vi "Setup.vi"(8 "error in (no error)":errorcluster, 11 "Setup Error In":refnum<class "Setup Error.lvclass">) -> (0 "error out":errorcluster, 3 "Setup Error Out":refnum<class "Setup Error.lvclass">)   [LabVIEW 2020, in "Setup Error.lvclass"]
doc: "Setup method called by the testing framework to set up test fixture before each test method is called."
uses:
  Setup Error.lvclass
  source/LUnit Test Case.lvclass
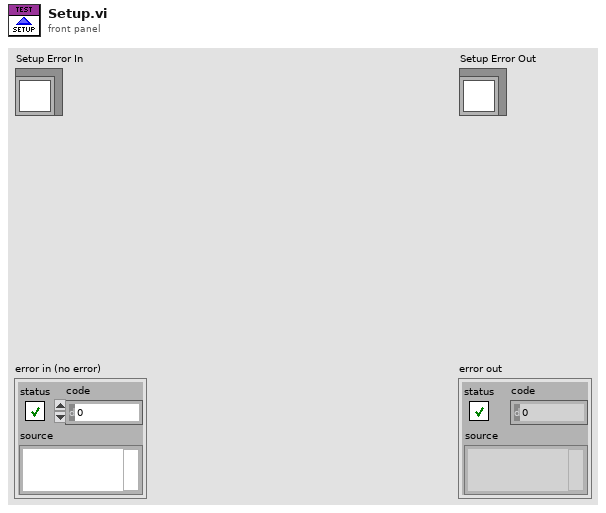
[diagram p1: front panel]
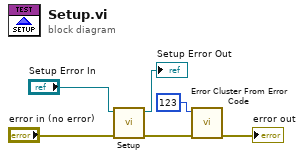
[diagram p0: block diagram]
diagram:
  n1 = call-parent "Setup.vi"("error in (no error)"="error in (no error)", "LUnit Test Case In"="Setup Error In") -> ("error out"=w6:errorcluster, "LUnit Test Case Out"=→"Setup Error Out":refnum<class "Setup Error.lvclass">)  [unwired: 8 in]
  n2 = call <vilib>:"Error Cluster From Error Code.vi"("error in (no error)"=w6, "error code (0)"=123) -> ("error out"=→"error out":errorcluster)  [unwired: 7 in]
